vi "Main.vi"() -> ()   [LabVIEW 2014, in "GenNet-Server.lvlib"]
doc: "The GenNet-Server module is instantiated from a DQMH Generic Networking Module\nin order to accept messages via TCP/IP. \n\nThe GenNet-Server module accepts messages from any DQMH Generic Networking \nModule running in another application and/or on another PC.\n\n<b>Note:</b> This VI was modified by the <b>Validate DQMH Module</b> tool to upgrade it to the DQMH 5.0 approach to destroying cloneable module event references.\n\n<b>Note:</b> This VI was modified by the <b>Validate DQMH Module</b> tool to have the module name be passed as the Additional Information parameter with an Error Reported broadcast.\n\n<b>Note:</b> This VI was modified by the <b>Validate DQMH Module</b> tool to call the Release Message Queue VI in the top-level Error case.\n\n<b>Note:</b> This VI was modified by the <b>Validate DQMH Module</b> tool to call the Release Message Queue VI in the top-level Error case."
uses:
  GenNet-Server.lvlib
  <vilib>/Delacor/Delacor QMH/Libraries/Cloneable Module Admin_class/Delacor_lib_QMH_Cloneable Module Admin.lvclass
  DQMH-GenNet Message Queue.lvclass
  TCP_Comm-States.ctl
  UDP Broadcasting/Generic Broadcasts.ctl
  hse-dqmh/Dynamic Requesters/Singleton/Status Updated Argument--cluster.ctl
  hse-dqmh/Dynamic Requesters/Singleton/Error Reported Argument--cluster.ctl
  hse-dqmh/Dynamic Requesters/Singleton/Get Module Execution Status Argument--cluster.ctl
  hse-dqmh/Dynamic Requesters/Singleton/Stop Argument--cluster.ctl
  hse-dqmh/Controls/System Message Argument--cluster.ctl
  hse-dqmh/Controls/System Message Source.ctl
  Module Data--cluster.ctl
  UDP Broadcasting/Network Broadcast Params.ctl
  Stop Argument--cluster.ctl
  <vilib>/Delacor/Delacor QMH/Libraries/Message Queue_class/Delacor_lib_QMH_Message Queue.lvclass/Delacor_lib_QMH_Message Queue.ctl
  UDP Broadcasting/Broadcast Arguments/Error Reported - Arguments.ctl
  UDP Broadcasting/Broadcast Arguments/Module Did Stop - Arguments.ctl
  Forward Generic Broadcasts to Network Argument--cluster.ctl
  <vilib>/Delacor/Delacor QMH/Libraries/Cloneable Module Admin_class/Delacor_lib_QMH_Cloneable Module Admin.lvclass/Delacor_lib_QMH_Cloneable Module Admin.ctl
  <vilib>/Delacor/Delacor QMH/Libraries/Module Admin_class/Delacor_lib_QMH_Module Admin.lvclass/Delacor_lib_QMH_Module Admin.ctl
  <vilib>/Utility/miscctls.llb/LVPointTypeDef.ctl
  <vilib>/Delacor/Delacor QMH/Libraries/Message Queue_class/Delacor_lib_QMH_Enqueue Message (Single).vi
  <vilib>/Delacor/Delacor QMH/Libraries/Cloneable Module Admin_class/Delacor_lib_QMH_Get Module ID.vi
  <vilib>/Delacor/Delacor QMH/Libraries/Module Admin_class/Delacor_lib_QMH_Get External Launch.vi
  <vilib>/Utility/tcp.llb/UDP Multicast Write-Only Open.vi
  <vilib>/Utility/error.llb/Error Cluster From Error Code.vi
  <vilib>/ErrorRing/Error Ring.xnode
  <vilib>/Delacor/Delacor QMH/Libraries/Message Queue_class/Delacor_lib_QMH_Message Queue.lvclass
  hse-dqmh/hse-dqmh.lvlib
  hse-gennet.lvlib
  hse-dqmh/hse-dqmh-dynamicrequesters.lvlib
panel:
  in  "Call Chain":string[](array[string])
  out "listener ID":refnum<k5>
  in  "Port Number":u16
  in  "Caller MsgQ":refnum<class "DQMH-GenNet Message Queue.lvclass">
  out "error out":errorcluster
  in  "Module Admin":refnum<class "Delacor_lib_QMH_Cloneable Module Admin.lvclass">
  # "The GenNet-Server module is instantiated from a DQMH Generic Networking Module\n(the caller) in order to accept messages via TCP/IP. \n\nThe GenNet-Server module accepts messages from any DQMH Generic Networking \nModule running in another application and/or on another PC."
  # "Caveat:\nThe Caller's message queue, which should be private to the caller only, is avail-\nable to the GenNet-Server module so that it can write messages directly. As the GenNet-Server\nmodule cannot be accessed from other code, and as messages that arrive via\nnetwork are to be considered local, this excemption to the rule is tolerable."
  # "Please get in touch with us at office@hampel-soft.com or visit our website www.hampel-soft.com"
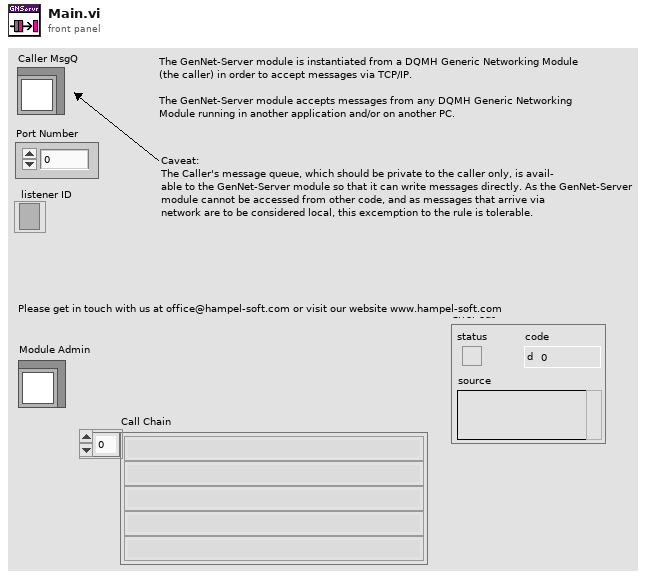
[diagram p1: front panel]
types:
  T1 = typedef "hse-gennet.lvlib/Generic Broadcasts.ctl" = cluster{"Status Updated":refnum<user-event>, "Error Reported":refnum<user-event>, "Update Module Execution Status":refnum<user-event>, "Module Did Stop":refnum<user-event>, "System Message":refnum<user-event>}
  T2 = typedef "GenNet-Server.lvlib/TCP_Comm-States.ctl" = enum16{"Idle", "Open port", "Wait for connection...", "Close port"}
  T3 = typedef "GenNet-Server.lvlib/Request Events--cluster.ctl" = cluster{"Stop Module":refnum<user-event>, "Show Panel":refnum<user-event>, "Hide Panel":refnum<user-event>, "Show Diagram":refnum<user-event>, "Get Module Execution Status":refnum<user-event>, "Forward Generic Broadcasts to Network":refnum<user-event>}
  T4 = typedef "GenNet-Server.lvlib/Module Data--cluster.ctl" = cluster{"Status":string, "UDP Conn. ID":refnum<k16>, "Network Broadcast Params":T5}
  T5 = typedef "hse-gennet.lvlib/Network Broadcast Params.ctl" = cluster{"Server (Sender) Port":u16, "Client (Receiver) Port":u16, "Multicast Address":string, "Local IP Address":string, "Max Rx Byte Size":i32}
  T6 = enum32{"invalid lock state", "Not Locked", "Locked (No Password)", "Password-protected"}
  T7 = typedef "GenNet-Server.lvlib/Stop Argument--cluster.ctl" = cluster{"Origin":string, "Module ID":i32, "Exit via Stop Module Req?":bool, "Wait for Module to stop?":bool}
  T8 = typedef "hse-gennet.lvlib/Error Reported - Arguments.ctl" = cluster{"Error":errorcluster, "Additional Information":string, "Module Name":string}
  T9 = typedef "hse-gennet.lvlib/Module Did Stop - Arguments.ctl" = cluster{"Origin":string, "Exit via Stop Module Req?":bool, "Wait for Module to stop?":bool}
  T10 = typedef "hse-dqmh.lvlib/System Message Source.ctl" = enum16{"module", "application", "network"}
  T11 = typedef "hse-dqmh.lvlib/System Message Argument--cluster.ctl" = cluster{"Identifier":string, "Payload":variant, "Source Type":T10, "Source Name":string}
  T12 = typedef "GenNet-Server.lvlib/Forward Generic Broadcasts to Network Argument--cluster.ctl" = cluster{"Module ID":i32, "Generic Broadcast Events":T1, "Network Broadcast Params":T5}
  T13 = typedef "LVPointTypeDef.ctl" = cluster{"Horizontal":i16, "Vertical":i16}
  T14 = enum32{"Invalid", "Standard", "Closed", "Hidden", "Minimized", "Maximized"}
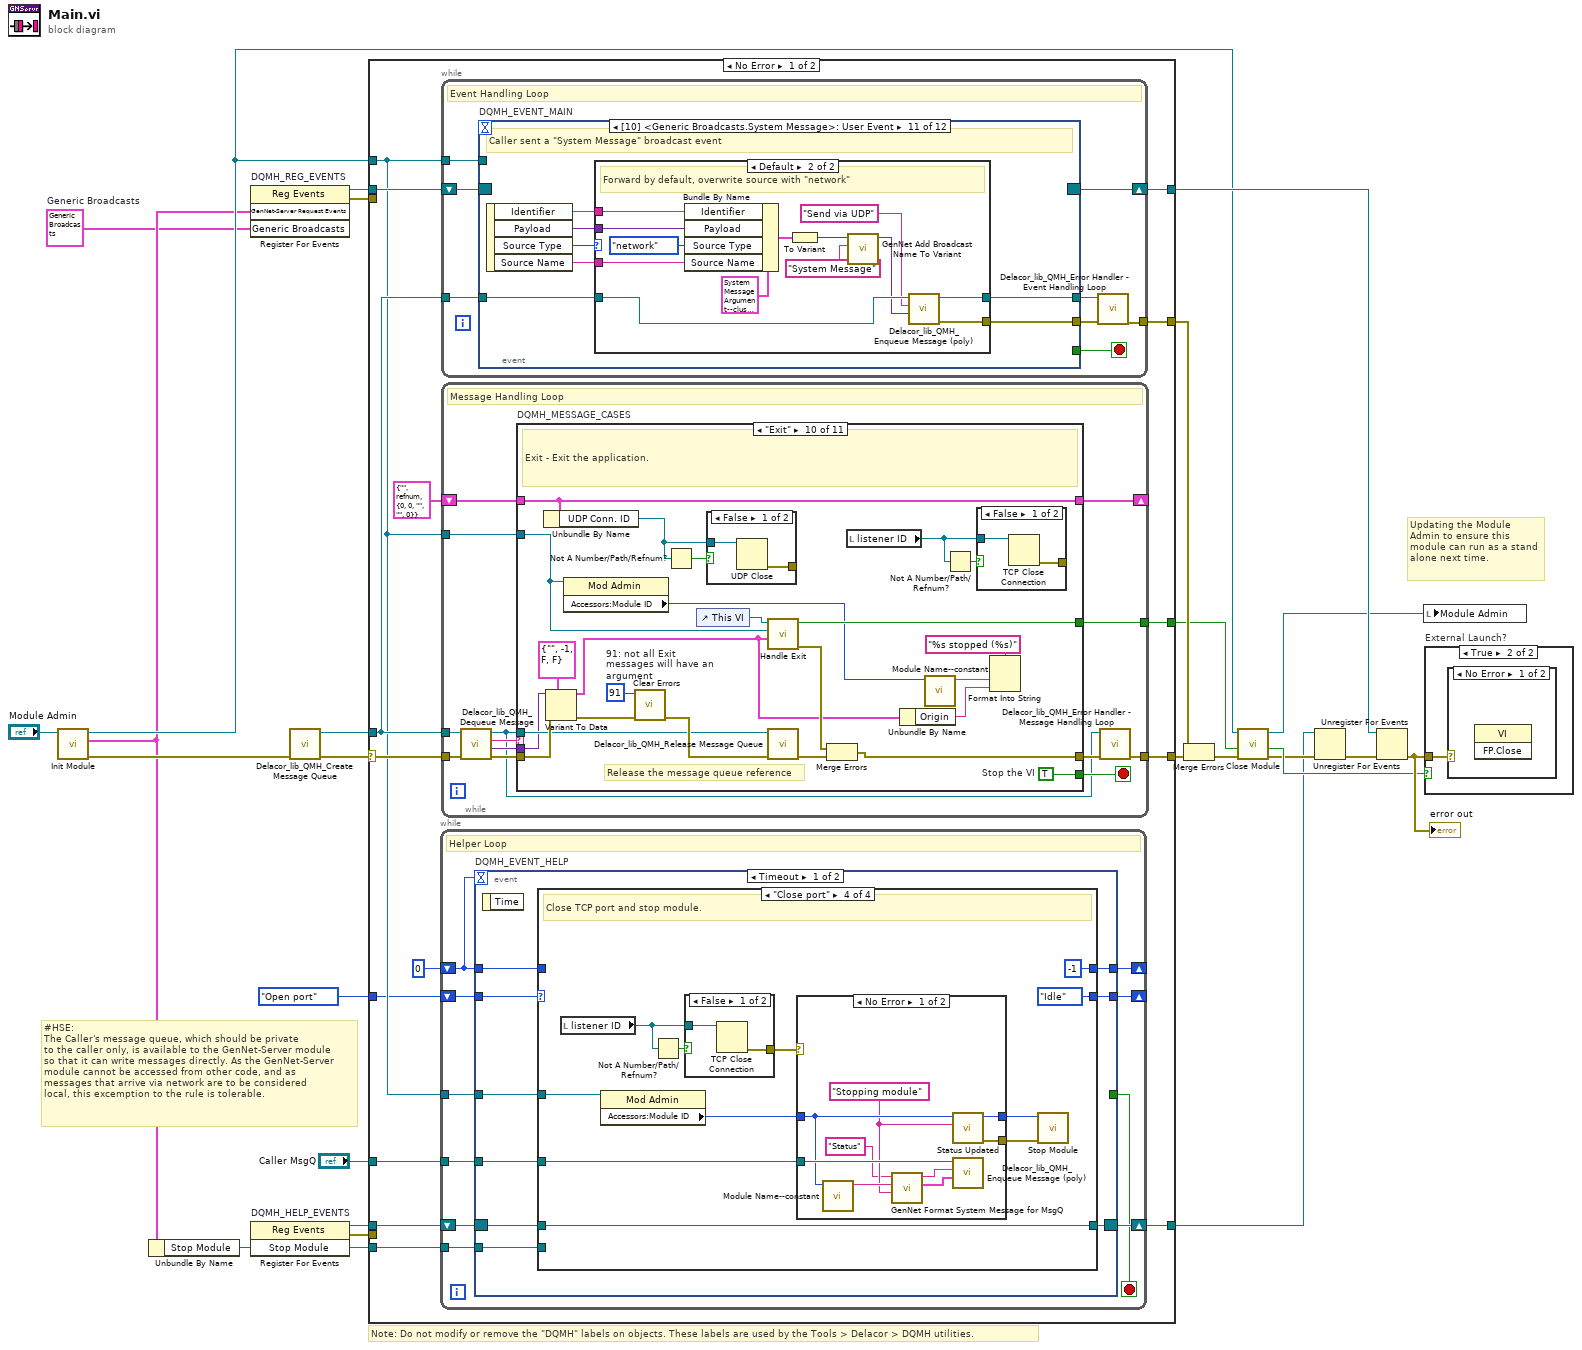
[diagram p0: block diagram]
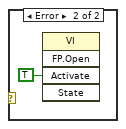
[diagram p3: hidden frame]
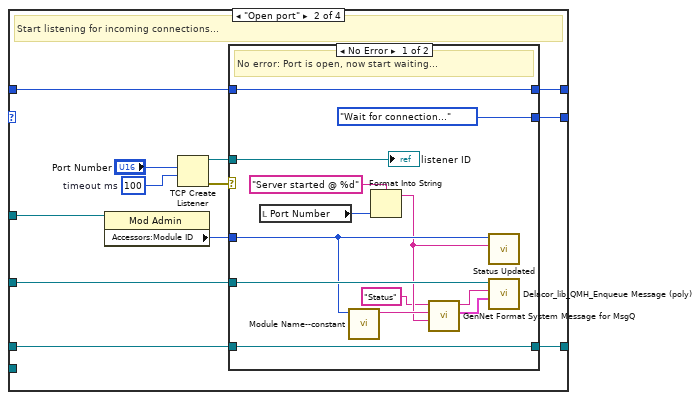
[diagram p5: hidden frame]
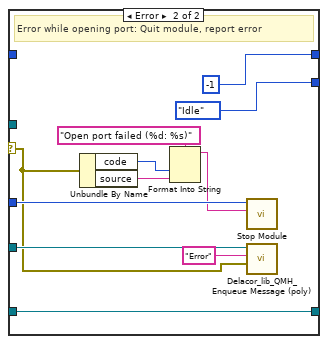
[diagram p6: hidden frame]
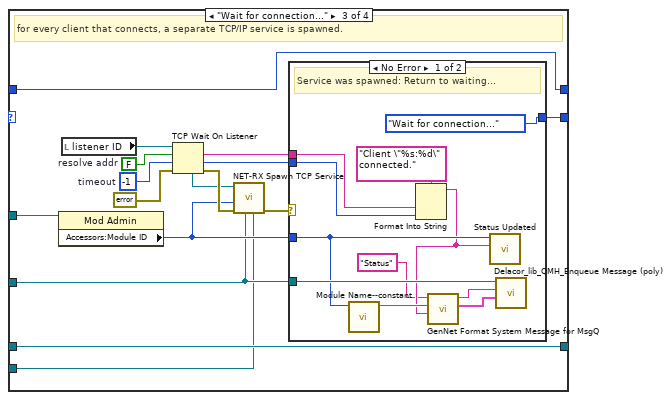
[diagram p7: hidden frame]
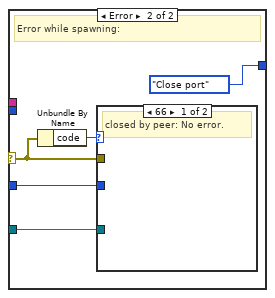
[diagram p8: hidden frame]
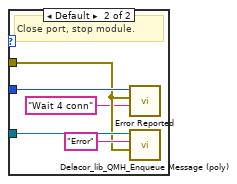
[diagram p9: hidden frame]
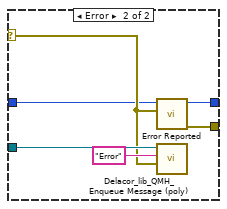
[diagram p11: hidden frame]
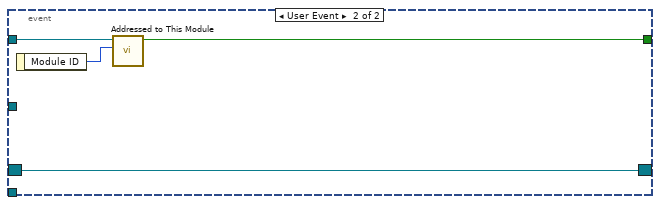
[diagram p12: hidden frame]
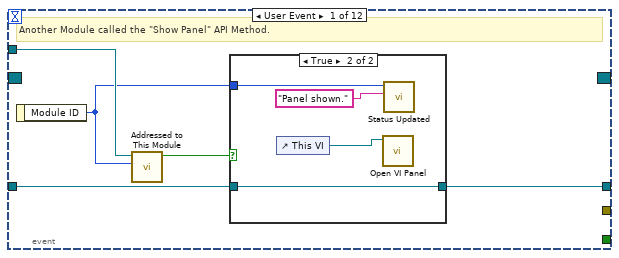
[diagram p13: hidden frame]
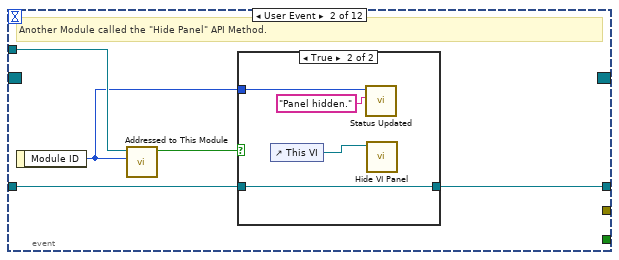
[diagram p15: hidden frame]
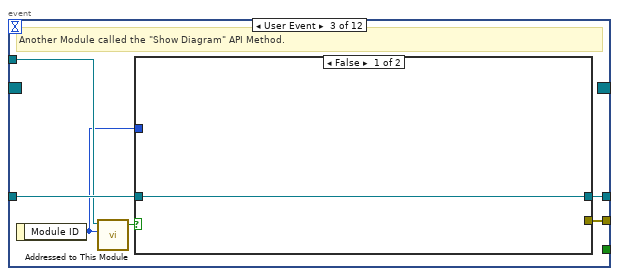
[diagram p17: hidden frame]
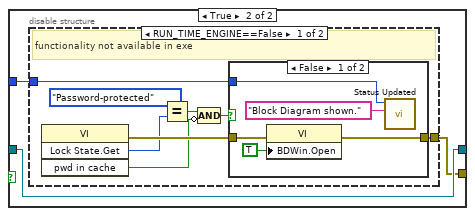
[diagram p18: hidden frame]
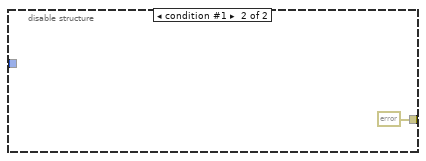
[diagram p20: hidden frame]
diagram:
  w1 = T1 {"Status Updated"=refnum, "Error Reported"=refnum, "Update Module Execution Status"=refnum, "Module Did Stop"=refnum, "System Message"=refnum}  # Generic Broadcasts
  # "#HSE: \nThe Caller's message queue, which should be private \nto the caller only, is available to the GenNet-Server module \nso that it can write messages directly. As the GenNet-Server\nmodule cannot be accessed from other code, and as \nmessages that arrive via network are to be considered \nlocal, this excemption to the rule is tolerable."
  # "Note: Do not modify or remove the \"DQMH\" labels on objects. These labels are used by the Tools > Delacor > DQMH utilities."
  # "Updating the Module Admin to ensure this module can run as a stand alone next time."
  n1 = call "Init Module.vi"("Cloneable Module Admin in"="Module Admin") -> ("error out"=w22:errorcluster, "GenNet-Server Request Events"=w6:T3, "Cloneable Module Admin out"=w17:refnum<class "Delacor_lib_QMH_Cloneable Module Admin.lvclass">)  [unwired: 8 in]
  n2 = Unbundle By Name(w6) -> ("Stop Module"=w5:refnum<user-event>)
  n3 = register-events "DQMH_REG_EVENTS"(w6, w1) -> (reference out=w20:refnum<event-registration>, error out=w3:errorcluster)  [unwired: 2 in]
  n4 = register-events "DQMH_HELP_EVENTS"(w5) -> (reference out=w11:refnum<event-registration>, error out=w2:errorcluster)  [unwired: 2 in]
  n5 = call <vilib>:"Delacor_lib_QMH_Create Message Queue.vi"("error in (no error)"=w22) -> ("error out"=w12:errorcluster, "Message Queue"=w19:refnum<class "Delacor_lib_QMH_Message Queue.lvclass">)  [unwired: 9 in]
  n6 = case shown="No Error" w12 {
    selector: w12 -> [w34 w500]
    tunnel: [w40 w500] -> w23
    tunnel: [w39 w501] -> w21
    tunnel: w20 -> [w37 w501]
    tunnel: w19 -> [w36 w492]
    tunnel: [w35 _] -> w24
    tunnel: w17 -> [w31 w496]
    tunnel: [w33 _] -> w15
    tunnel: w11 -> [w32 w493]
    tunnel: "Caller MsgQ" -> [w30 w491]
    tunnel: [w29 w493] -> w7
    tunnel: w5 -> [w27 _]
    tunnel: TCP_Comm-States."Open port" ("comm-states") -> [w26 _]
    tunnel: w3 -> [_ _]
    tunnel: w2 -> [_ _]
    frame No Error {
      n7 = while {
        shift-right: [w49] -> _
        shift-left: 0 -> [w50]
        tunnel: w31 -> [w48]
        tunnel: w30 -> [w47]
        shift-right: [w44] -> _
        shift-left: w26 -> [w45]
        shift-right: [w46] -> w29
        shift-left: w32 -> [w42]
        tunnel: w27 -> [w41]
        stop <- w43 stop-if-true
        # "Helper Loop"
        n8 = event "DQMH_EVENT_HELP" shown="[0] Timeout" {
          selector: w42 -> [w53 w162]
          dyn-events: [w52 w162] -> w46
          timeout: w50 -> [_ _]
          tunnel: w50 -> [w58 _]
          tunnel: [w57 _] -> w49
          tunnel: w48 -> [w56 w165]
          tunnel: w47 -> [w54 _]
          tunnel: w45 -> [w59 _]
          tunnel: [w55 _] -> w44
          tunnel: [_ w163] -> w43
          tunnel: w41 -> [w51 _]
          event Timeout {
            n9 = event-data() -> ()  [unwired: 1 in, 1 out]
            n10 = case shown="\"Close port\"" w59 {
              selector: w59 -> [w62 _ _ _]
              tunnel: w58 -> [w61 w67 w99 _]
              tunnel: [w61 w66 w99 -1] -> w57
              tunnel: w56 -> [_ w70 w111 w145]
              tunnel: [w62 w74 w106 TCP_Comm-States."Idle" ("comm-states")] -> w55
              tunnel: w54 -> [_ w68 w107 w146]
              tunnel: w53 -> [w60 w65 w105 w139]
              tunnel: [w60 w64 w105 w139] -> w52
              tunnel: w51 -> [_ _ w104 _]
              frame "Idle", Default {
              }
              frame "Open port" {
                w73 = 100  # timeout ms
                # "Start listening for incoming connections..."
                n11 = property class="Mod Admin"(reference=w70) -> ("Accessors:Module ID"=w69:i32)  [unwired: 1 in, 2 out]
                n12 = TCP Create Listener(9:w73, 10:"Port Number") -> (0:w72:errorcluster, 3:w71:refnum<k5>)  [unwired: 3 in, 1 out]
                n13 = case shown="No Error" w72 {
                  selector: w72 -> [_ w88]
                  tunnel: [TCP_Comm-States."Wait for connection..." ("comm-states") TCP_Comm-States."Idle" ("comm-states")] -> w74
                  tunnel: w71 -> [w83 _]
                  tunnel: w69 -> [w78 w93]
                  tunnel: w68 -> [w85 w96]
                  tunnel: w67 -> [w84 _]
                  tunnel: [w84 -1] -> w66
                  tunnel: w65 -> [w82 w94]
                  tunnel: [w82 w94] -> w64
                  frame No Error {
                    # "No error: Port is open, now start waiting..."
                    n14 = local read "Port Number"() -> (w80:u16)
                    n15 = call "Module Name--constant.vi"("Module ID"=w78) -> ("Module Name"=w77:string)  [unwired: 10 in]
                    n16 = Format Into String(format string="Server started @ %d" ("Status"), w80) -> (resulting string=w76:string)  [unwired: 2 in, 1 out]
                    n17 = call "GenNet Format System Message for MsgQ.vi"("Payload"=w76, "Source Name"=w77, "Identifer"="Status") -> ("System Message Argument"=w79:T11, "System Message constant"=w87:string)  [unwired: 7 in]
                    n18 = call "Status Updated.vi"("Status"=w76, "Module ID"=w78) -> ()  [unwired: 9 in, 1 out]
                    n19 = call-poly <vilib>:"Delacor_lib_QMH_Enqueue Message (poly).vi"("Message Data"=w79, "Message"=w87, "Message Queue in"=w85) -> ()  [unwired: 7 in, 2 out]
                    "listener ID" <- w83
                  }
                  frame Error {
                    # "Error while opening port: Quit module, report error"
                    n20 = Unbundle By Name(w88) -> ("code"=w90:i32, "source"=w91:string)
                    n21 = Format Into String(format string="Open port failed (%d: %s)" ("Origin"), w90, w91) -> (resulting string=w89:string)  [unwired: 2 in, 1 out]
                    n22 = call "Stop Module.vi"("Origin"=w89, "Module ID"=w93) -> ()  [unwired: 9 in, 1 out]
                    n23 = call-poly <vilib>:"Delacor_lib_QMH_Enqueue Message (poly).vi"("Message Data"=w88, "Message"="Error", "Message Queue in"=w96) -> ()  [unwired: 7 in, 2 out]
                  }
                }
              }
              frame "Wait for connection..." {
                w101 = FALSE  # resolve addr
                w114 = -1  # timeout
                # "for every client that connects, a separate TCP/IP service is spawned."
                n24 = property class="Mod Admin"(reference=w111) -> ("Accessors:Module ID"=w109:i32)  [unwired: 1 in, 2 out]
                n25 = local read "listener ID"() -> (w108:refnum<k5>)
                n26 = TCP Wait On Listener(8:errorcluster {"status"=FALSE, "code"=0, "source"=""} ("error in (no error)"), 9:w114, 10:w101, 11:w108) -> (0:w113:errorcluster, 1:w102:u16, 2:w103:string, 4:w112:refnum<k5>)  [unwired: 1 out]
                n27 = call "NET-RX Spawn TCP Service.vi"("Stop Module"=w104, "Caller MsgQ"=w107, "error in"=w113, "Module ID"=w109, "Connection ID"=w112) -> ("error out"=w110:errorcluster)  [unwired: 6 in]
                n28 = case shown="No Error" w110 {
                  selector: w110 -> [_ w127]
                  tunnel: w107 -> [w121 w130]
                  tunnel: w109 -> [w118 w129]
                  tunnel: [TCP_Comm-States."Wait for connection..." ("comm-states") TCP_Comm-States."Close port" ("comm-states")] -> w106
                  tunnel: w103 -> [w123 _]
                  tunnel: w102 -> [w122 _]
                  frame No Error {
                    # "Service was spawned: Return to waiting..."
                    n29 = call "Module Name--constant.vi"("Module ID"=w118) -> ("Module Name"=w117:string)  [unwired: 10 in]
                    n30 = Format Into String(format string="Client \"%s:%d\" connected.", w123, w122) -> (resulting string=w116:string)  [unwired: 2 in, 1 out]
                    n31 = call "GenNet Format System Message for MsgQ.vi"("Payload"=w116, "Source Name"=w117, "Identifer"="Status") -> ("System Message Argument"=w120:T11, "System Message constant"=w119:string)  [unwired: 7 in]
                    n32 = call "Status Updated.vi"("Status"=w116, "Module ID"=w118) -> ()  [unwired: 9 in, 1 out]
                    n33 = call-poly <vilib>:"Delacor_lib_QMH_Enqueue Message (poly).vi"("Message Data"=w120, "Message"=w119, "Message Queue in"=w121) -> ()  [unwired: 7 in, 2 out]
                  }
                  frame Error {
                    # "Error while spawning:"
                    n34 = Unbundle By Name(w127) -> ("code"=w126:i32)
                    n35 = case shown="66" w126 {
                      tunnel: w130 -> [_ w135]
                      tunnel: w127 -> [_ w132]
                      tunnel: w129 -> [_ w133]
                      frame 66 {
                        # "closed by peer: No error."
                      }
                      frame Default {
                        # "Close port, stop module."
                        n36 = call "Error Reported.vi"("Additional Information"="Wait 4 conn", "Error"=w132, "Module ID"=w133) -> ()  [unwired: 8 in, 1 out]
                        n37 = call-poly <vilib>:"Delacor_lib_QMH_Enqueue Message (poly).vi"("Message Data"=w132, "Message"="Error", "Message Queue in"=w135) -> ()  [unwired: 7 in, 2 out]
                      }
                    }
                  }
                }
              }
              frame "Close port" {
                # "Close TCP port and stop module."
                n38 = local read "listener ID"() -> (w140:refnum<k5>)
                n39 = property class="Mod Admin"(reference=w145) -> ("Accessors:Module ID"=w138:i32)  [unwired: 1 in, 2 out]
                n40 = Not A Number/Path/Refnum?(number/path/refnum=w140) -> (NaN/Path/Refnum?=w142:bool)
                n41 = case shown="False" w142 {
                  tunnel: [w148 _] -> w141
                  tunnel: w140 -> [w147 _]
                  frame False {
                    n42 = TCP Close Connection(connection ID=w147) -> (error out=w148:errorcluster)  [unwired: 2 in, 1 out]
                  }
                  frame True {
                  }
                }
                n43 = case shown="No Error" w141 {
                  selector: w141 -> [_ w159]
                  tunnel: w146 -> [w155 w160]
                  tunnel: w138 -> [w152 w157]
                  tunnel: [w156 w158] -> w137
                  tunnel: [w152 w157] -> w136
                  frame No Error {
                    w150 = "Stopping module" ("Status")
                    n44 = call "Module Name--constant.vi"("Module ID"=w152) -> ("Module Name"=w151:string)  [unwired: 10 in]
                    n45 = call "GenNet Format System Message for MsgQ.vi"("Payload"=w150, "Source Name"=w151, "Identifer"="Status") -> ("System Message Argument"=w153:T11, "System Message constant"=w154:string)  [unwired: 7 in]
                    n46 = call "Status Updated.vi"("Status"=w150, "Module ID"=w152) -> ("error out"=w156:errorcluster)  [unwired: 9 in]
                    n47 = call-poly <vilib>:"Delacor_lib_QMH_Enqueue Message (poly).vi"("Message Data"=w153, "Message"=w154, "Message Queue in"=w155) -> ()  [unwired: 7 in, 2 out]
                  }
                  frame Error {
                    n48 = call "Error Reported.vi"("Error"=w159, "Module ID"=w157) -> ("error out"=w158:errorcluster)  [unwired: 9 in]
                    n49 = call-poly <vilib>:"Delacor_lib_QMH_Enqueue Message (poly).vi"("Message Data"=w159, "Message"="Error", "Message Queue in"=w160) -> ()  [unwired: 7 in, 2 out]
                  }
                }
                n50 = call "Stop Module.vi"("error in (no error)"=w137, "Module ID"=w136) -> ()  [unwired: 9 in, 1 out]
              }
            }
          }
          event User Event {
            n51 = event-data() -> ("Module ID"=w164:i32)  [unwired: 1 in]
            n52 = call "Addressed to This Module.vi"("Module ID from Argument"=w164, "Module Admin"=w165) -> ("Addressed to this instance?"=w163:bool)  [unwired: 8 in, 1 out]
          }
        }
      }
      n53 = while {
        tunnel: w36 -> [w173]
        shift-right: [w171] -> w39
        shift-left: w37 -> [w172]
        tunnel: [w167] -> w35
        tunnel: w31 -> [w166]
        stop <- w169 stop-if-true
        # "Event Handling Loop"
        n54 = event "DQMH_EVENT_MAIN" shown="[10] <Generic Broadcasts.System Message>: User Event" {
          selector: w172 -> [_ _ _ _ _ _ _ _ _ _ _ w318]
          dyn-events: [_ _ _ _ _ _ _ _ _ _ _ w319] -> w171
          timeout: _ -> [_ _ _ _ _ _ _ _ _ _ _ _]
          tunnel: [_ _ _ w222 _ _ _ _ _ _ _ _] -> w169
          tunnel: w173 -> [w178 w188 w199 w225 w245 w249 w261 w274 w280 w293 w301 w325]
          tunnel: [_ _ w194 w227 w244 w248 w259 w271 w279 w291 w299 w321] -> w170
          tunnel: [w177 w187 w198 w226 w243 w249 w260 w272 w281 w292 w300 w324] -> w168
          tunnel: w166 -> [w175 w185 w196 w224 _ w250 _ _ _ _ _ w322]
          event User Event {
            # "Another Module called the \"Show Panel\" API Method."
            n55 = event-data() -> ("Module ID"=w174:i32)  [unwired: 1 in]
            n56 = call "Addressed to This Module.vi"("Module ID from Argument"=w174, "Module Admin"=w175) -> ("Addressed to this instance?"=w176:bool)  [unwired: 8 in, 1 out]
            n57 = case shown="True" w176 {
              tunnel: w178 -> [w179 w183]
              tunnel: [w179 w183] -> w177
              tunnel: w174 -> [_ w181]
              frame False {
              }
              frame True {
                n58 = control-ref of="This VI"() -> (w180:refnum<vi>)
                n59 = call "Open VI Panel.vi"("VI"=w180) -> ()  [unwired: 10 in, 1 out]
                n60 = call "Status Updated.vi"("Status"="Panel shown." ("format string"), "Module ID"=w181) -> ()  [unwired: 9 in, 1 out]
              }
            }
          }
          event User Event {
            # "Another Module called the \"Hide Panel\" API Method."
            n61 = event-data() -> ("Module ID"=w184:i32)  [unwired: 1 in]
            n62 = call "Addressed to This Module.vi"("Module ID from Argument"=w184, "Module Admin"=w185) -> ("Addressed to this instance?"=w186:bool)  [unwired: 8 in, 1 out]
            n63 = case shown="True" w186 {
              tunnel: w188 -> [w189 w193]
              tunnel: [w189 w193] -> w187
              tunnel: w184 -> [_ w191]
              frame False {
              }
              frame True {
                n64 = control-ref of="This VI"() -> (w190:refnum<vi>)
                n65 = call "Status Updated.vi"("Status"="Panel hidden." ("format string"), "Module ID"=w191) -> ()  [unwired: 9 in, 1 out]
                n66 = call "Hide VI Panel.vi"("VI"=w190) -> ()  [unwired: 10 in, 1 out]
              }
            }
          }
          event User Event {
            # "Another Module called the \"Show Diagram\" API Method."
            n67 = event-data() -> ("Module ID"=w195:i32)  [unwired: 1 in]
            n68 = call "Addressed to This Module.vi"("Module ID from Argument"=w195, "Module Admin"=w196) -> ("Addressed to this instance?"=w197:bool)  [unwired: 8 in, 1 out]
            n69 = case shown="False" w197 {
              tunnel: w199 -> [w200 w202]
              tunnel: [w200 w202] -> w198
              tunnel: w195 -> [_ w203]
              tunnel: [_ w201] -> w194
              frame False {
              }
              frame True {
                n70 = disable-structure shown="RUN_TIME_ENGINE==False" {
                  disable-tunnel: [w211 errorcluster {"status"=FALSE, "code"=0, "source"=""} ("error out")] -> w201
                  disable-tunnel: w203 -> [w204 _]
                  frame condition #0 (active) {
                    # "functionality not available in exe"
                    n71 = invoke class="VI" method="Lock State.Get"() -> (error out=w210:errorcluster, "Get Lock State"=w209:T6, "pwd in cache"=w206:bool)  [unwired: 4 in, 1 out]
                    n72 = Equal?(x=T6."Password-protected", y=w209) -> (x = y?=w207:bool)
                    n73 = Compound Arithmetic op=AND(w207, invert w206) -> (w205:bool)
                    n74 = case shown="False" w205 {
                      tunnel: [w215 w217] -> w211
                      tunnel: w210 -> [w214 w217]
                      tunnel: w204 -> [w212 _]
                      frame False {
                        n75 = property class="VI"(error in=w214, "BDWin.Open"=TRUE ("Block Diagram Window:Open")) -> (error out=w215:errorcluster)  [unwired: 1 in, 1 out]
                        n76 = call "Status Updated.vi"("Status"="Block Diagram shown." ("format string"), "Module ID"=w212) -> ()  [unwired: 9 in, 1 out]
                      }
                      frame True {
                        # "Password-protected VI, and the password is not in the cache. Do not show the diagram."
                      }
                    }
                  }
                  frame condition #1 {
                  }
                }
              }
            }
          }
          event User Event {
            # "Another Module called the \"Stop Module\" API Method  or the Message Handling Loop below."
            n77 = event-data() -> ("Module ID"=w220:i32, "Wait for Module to stop?"=w221:bool, "Origin"=w219:string)  [unwired: 1 in]
            n78 = call "Addressed to This Module.vi"("Module ID from Argument"=w220, "Module Admin"=w224) -> ("Addressed to this instance?"=w223:bool)  [unwired: 8 in, 1 out]
            n79 = case shown="True" w223 {
              tunnel: [_ w237] -> w227
              tunnel: [w228 w236] -> w226
              tunnel: w225 -> [w228 w235]
              tunnel: [_ TRUE] -> w222
              tunnel: w221 -> [_ w230]
              tunnel: w220 -> [_ w232]
              tunnel: w219 -> [_ _]
              frame False {
              }
              frame True {
                # "The event can get fired from the Exit message. The queue gets destroyed there. In this case, the Enqueue VI will return error 1. It is safe to ignore, because the module is already exiting."
                n80 = Bundle By Name(cluster=T7 {"Origin"="", "Module ID"=-1, "Exit via Stop Module Req?"=FALSE, "Wait for Module to stop?"=FALSE} ("Stop Argument"), "Module ID"=w232, "Exit via Stop Module Req?"=TRUE, "Wait for Module to stop?"=w230) -> (w229:T7)
                n81 = call-poly <vilib>:"Delacor_lib_QMH_Enqueue Message (poly).vi"("Priority Message? (F)"=TRUE, "Message Data"=w229, "Message"="Exit", "Message Queue in"=w235) -> ("error out"=w240:errorcluster, "Message Queue out"=w236:refnum<class "Delacor_lib_QMH_Message Queue.lvclass">)  [unwired: 6 in]
                n82 = call <vilib>:"Clear Errors.vi"("error in (no error)"=w240, "specific error code to clear (0: all)"=1) -> ("error out"=w237:errorcluster)  [unwired: 4 in, 1 out]
              }
            }
          }
          event Panel Close? {
            w246 = TRUE  # Discard the event so the 'Confirm Quit' message has a chance to run.
            # "Send the 'Confirm Quit' message if the user closes the panel of the VI."
            n83 = event-data() -> ()  [unwired: 1 in, 1 out]
            n84 = call-poly <vilib>:"Delacor_lib_QMH_Enqueue Message (poly).vi"("Message"="Confirm Quit", "Message Queue in"=w245) -> ("error out"=w244:errorcluster, "Message Queue out"=w243:refnum<class "Delacor_lib_QMH_Message Queue.lvclass">)  [unwired: 8 in]
            n85 = event-data("Discard?"=w246) -> ()  [unwired: 1 in, 1 out]
          }
          event User Event {
            # "For cloneable running as singleton, broadcast that the module is running."
            n86 = event-data() -> ("Module ID"=w247:i32)  [unwired: 1 in]
            n87 = call "Addressed to This Module.vi"("Module ID from Argument"=w247, "Module Admin"=w250) -> ("Addressed to this instance?"=w251:bool)  [unwired: 8 in, 1 out]
            n88 = case shown="True" w251 {
              tunnel: [_ w254] -> w248
              tunnel: w247 -> [_ w253]
              frame False {
              }
              frame True {
                n89 = call "Update Module Execution Status.vi"("Running?"=TRUE, "Module ID"=w253) -> ("error out"=w254:errorcluster)  [unwired: 9 in]
              }
            }
          }
          event User Event {
            # "Caller sent a \"Status Updated\" broadcast event"
            n90 = event-data() -> ("Status"=w256:string)  [unwired: 1 in]
            n91 = To Variant(anything=w256) -> (Variant=w258:variant)
            n92 = call "GenNet Add Broadcast Name To Variant.vi"("Broadcast Name"="Status Updated", "Broadcast Data IN"=w258) -> ("Variant OUT"=w255:variant)  [unwired: 9 in]
            n93 = call-poly <vilib>:"Delacor_lib_QMH_Enqueue Message (poly).vi"("Message Data"=w255, "Message"="Send via UDP", "Message Queue in"=w261) -> ("error out"=w259:errorcluster, "Message Queue out"=w260:refnum<class "Delacor_lib_QMH_Message Queue.lvclass">)  [unwired: 7 in]
          }
          event User Event {
            # "Caller sent a \"Error reported\" broadcast event"
            n94 = event-data() -> ("Error"=w269:errorcluster, "Additional Information"=w268:string, "Module Name"=w267:string)  [unwired: 1 in]
            n95 = Bundle By Name(cluster=T8 {"Error"={"status"=FALSE, "code"=0, "source"=""}, "Additional Information"="", "Module Name"=""}, "Error"=w269, "Additional Information"=w268, "Module Name"=w267) -> (w264:T8)
            n96 = To Variant(anything=w264) -> (Variant=w266:variant)
            n97 = call "GenNet Add Broadcast Name To Variant.vi"("Broadcast Name"="Error Reported", "Broadcast Data IN"=w266) -> ("Variant OUT"=w263:variant)  [unwired: 9 in]
            n98 = call-poly <vilib>:"Delacor_lib_QMH_Enqueue Message (poly).vi"("Message Data"=w263, "Message"="Send via UDP", "Message Queue in"=w274) -> ("error out"=w271:errorcluster, "Message Queue out"=w272:refnum<class "Delacor_lib_QMH_Message Queue.lvclass">)  [unwired: 7 in]
          }
          event User Event {
            # "Caller sent a \"Update Module Execution Status\" broadcast event"
            n99 = event-data() -> ("Running?"=w276:bool)  [unwired: 1 in]
            n100 = To Variant(anything=w276) -> (Variant=w278:variant)
            n101 = call "GenNet Add Broadcast Name To Variant.vi"("Broadcast Name"="Update Module Execution Status", "Broadcast Data IN"=w278) -> ("Variant OUT"=w275:variant)  [unwired: 9 in]
            n102 = call-poly <vilib>:"Delacor_lib_QMH_Enqueue Message (poly).vi"("Message Data"=w275, "Message"="Send via UDP", "Message Queue in"=w280) -> ("error out"=w279:errorcluster, "Message Queue out"=w281:refnum<class "Delacor_lib_QMH_Message Queue.lvclass">)  [unwired: 7 in]
          }
          event User Event {
            # "Caller sent a \"Module Did Stop\" broadcast event"
            n103 = event-data() -> ("Origin"=w290:string, "Exit via Stop Module Req?"=w288:bool, "Wait for Module to stop?"=w289:bool)  [unwired: 1 in]
            n104 = Bundle By Name(cluster=T9 {"Origin"="", "Exit via Stop Module Req?"=FALSE, "Wait for Module to stop?"=FALSE} ("Module Did Stop - Arguments"), "Origin"=w290, "Exit via Stop Module Req?"=w288, "Wait for Module to stop?"=w289) -> (w284:T9)
            n105 = To Variant(anything=w284) -> (Variant=w287:variant)
            n106 = call "GenNet Add Broadcast Name To Variant.vi"("Broadcast Name"="Module Did Stop", "Broadcast Data IN"=w287) -> ("Variant OUT"=w283:variant)  [unwired: 9 in]
            n107 = call-poly <vilib>:"Delacor_lib_QMH_Enqueue Message (poly).vi"("Message Data"=w283, "Message"="Send via UDP", "Message Queue in"=w293) -> ("error out"=w291:errorcluster, "Message Queue out"=w292:refnum<class "Delacor_lib_QMH_Message Queue.lvclass">)  [unwired: 7 in]
          }
          event User Event {
            # "Caller sent a \"System Message\" broadcast event"
            n108 = event-data() -> ("Identifier"=w298:string, "Payload"=w297:variant, "Source Type"=w296:T10, "Source Name"=w295:string)  [unwired: 1 in]
            n109 = case shown="Default" w296 {
              tunnel: w301 -> [w302 w315]
              tunnel: [w302 w313] -> w300
              tunnel: [_ w312] -> w299
              tunnel: w298 -> [_ w311]
              tunnel: w297 -> [_ w310]
              tunnel: w295 -> [_ w304]
              frame "network" {
                # "Do not forward if originally received via network"
              }
              frame Default {
                # "Forward by default, overwrite source with \"network\""
                n110 = Bundle By Name(cluster=T11 {"Identifier"="", "Payload"=variant, "Source Type"=enum."module", "Source Name"=""} ("System Message Argument"), "Identifier"=w311, "Payload"=w310, "Source Type"=System_Message_Source."network" ("Source"), "Source Name"=w304) -> (w309:T11)
                n111 = To Variant(anything=w309) -> (Variant=w308:variant)
                n112 = call "GenNet Add Broadcast Name To Variant.vi"("Broadcast Name"="System Message", "Broadcast Data IN"=w308) -> ("Variant OUT"=w307:variant)  [unwired: 9 in]
                n113 = call-poly <vilib>:"Delacor_lib_QMH_Enqueue Message (poly).vi"("Message Data"=w307, "Message"="Send via UDP", "Message Queue in"=w315) -> ("error out"=w312:errorcluster, "Message Queue out"=w313:refnum<class "Delacor_lib_QMH_Message Queue.lvclass">)  [unwired: 7 in]
              }
            }
          }
          event User Event {
            # "Another Module called the \"Forward Generic Broadcasts to Network\" API Method."
            n114 = event-data() -> ("Generic Broadcast Events"=w317:T1, "Network Broadcast Params"=w316:T5, "Module ID"=w320:i32)  [unwired: 1 in]
            n115 = call "Addressed to This Module.vi"("Module ID from Argument"=w320, "Module Admin"=w322) -> ("Addressed to this instance?"=w323:bool)  [unwired: 8 in, 1 out]
            n116 = case shown="True" w323 {
              tunnel: w325 -> [w327 w337]
              tunnel: [w327 w336] -> w324
              tunnel: [_ w334] -> w321
              tunnel: [w326 w333] -> w319
              tunnel: w318 -> [w326 w332]
              tunnel: w317 -> [_ w331]
              tunnel: w316 -> [_ w330]
              frame False {
              }
              frame True {
                n117 = Bundle By Name(cluster=T12 {"Module ID"=-1, "Generic Broadcast Events"={"Status Updated"=refnum, "Error Reported"=refnum, "Update Module Execution Status"=refnum, "Module Did Stop"=refnum, "System Message"=refnum}, "Network Broadcast Params"={"Server (Sender) Port"=0, "Client (Receiver) Port"=0, "Multicast Address"="", "Local IP Address"="", "Max Rx Byte Size"=0}} ("Forward Generic Broadcasts to Network Argument"), "Network Broadcast Params"=w330) -> (w329:T12)
                n118 = register-events "DQMH_REG_INNER"(reference=w332, w331) -> (reference out=w333:refnum<event-registration>)  [unwired: 2 in, 1 out]
                n119 = call-poly <vilib>:"Delacor_lib_QMH_Enqueue Message (poly).vi"("Message Data"=w329, "Message"="Create UDP Sender", "Message Queue in"=w337) -> ("error out"=w334:errorcluster, "Message Queue out"=w336:refnum<class "Delacor_lib_QMH_Message Queue.lvclass">)  [unwired: 7 in]
              }
            }
          }
        }
        n120 = call-dynamic "Delacor_lib_QMH_Error Handler - Event Handling Loop.vi"("error in (no error)"=w170, "Message Queue in"=w168) -> ("dup error in"=w167:errorcluster)  [unwired: 8 in, 1 out]
      }
      n121 = while {
        tunnel: w36 -> [w342]
        shift-right: [w348] -> _
        shift-left: T4 {"Status"="", "UDP Conn. ID"=refnum, "Network Broadcast Params"={"Server (Sender) Port"=0, "Client (Receiver) Port"=0, "Multicast Address"="", "Local IP Address"="", "Max Rx Byte Size"=0}} ("Data Cluster") -> [w349]
        tunnel: w34 -> [w346]
        tunnel: [w340] -> w40
        tunnel: w31 -> [w339]
        tunnel: [w338] -> w33
        stop <- w347 stop-if-true
        # "Message Handling Loop"
        n122 = call-dynamic "Delacor_lib_QMH_Dequeue Message.vi"("error in (no error)"=w346, "Message Queue in"=w342) -> ("error out"=w345:errorcluster, "Message Data"=w343:variant, "Message"=w344:string, "Message Queue out"=w341:refnum<class "Delacor_lib_QMH_Message Queue.lvclass">)  [unwired: 6 in]
        n123 = case "DQMH_MESSAGE_CASES" shown="\"Exit\"" w344 {
          selector: w344 -> [_ _ _ _ _ _ _ _ _ _ w480]
          tunnel: w341 -> [_ _ _ _ _ _ _ w427 w445 w470 _]
          tunnel: w345 -> [w366 w379 w386 w401 w417 w420 w423 w436 w444 w472 _]
          tunnel: [w351 w377 w394 w403 w415 w418 w421 w426 w443 w449 w481] -> w350
          tunnel: w349 -> [w365 w378 w392 w402 w416 w419 w422 w435 w448 w451 w482]
          tunnel: [w365 w378 w391 w402 w416 w419 w422 w435 w448 w451 w482] -> w348
          tunnel: [_ _ _ _ _ _ _ _ _ w469 _] -> w347
          tunnel: w343 -> [_ _ w384 w400 _ _ _ w434 _ w464 _]
          tunnel: w339 -> [w361 _ _ _ _ _ _ w431 _ w454 w478]
          tunnel: [_ _ _ _ _ _ _ _ _ w462 _] -> w338
          frame "Initialize" {
            # "\"Create UDP Sender\""
            # "Initialize - Any operation that needs to be done before the module can receive messages. Synchronize Caller Events.vi will inform Start Module.vi that the module has launched and is ready to receive messages. Module Did Init.vi will broadcast that the module initialized."
            n124 = call "Synchronize Caller Events.vi"("error in (no error)"=w366, "Module Admin"=w361) -> ("error out"=w363:errorcluster, "Module Admin out"=w360:refnum<class "Delacor_lib_QMH_Cloneable Module Admin.lvclass">)  [unwired: 8 in]
            n125 = property class="Mod Admin"(reference=w360) -> ("Accessors:Module ID"=w359:i32, "Accessors:External Launch"=w362:bool)  [unwired: 1 in, 2 out]
            n126 = call "Module Name--constant.vi"("Module ID"=w359) -> ("Module Name"=w352:string)  [unwired: 10 in]
            n127 = disable-structure shown="TARGET_TYPE==Windows||EMBEDDED_UI==True" {
              disable-tunnel: w362 -> [w369 _]
              disable-tunnel: w352 -> [w367 _]
              frame condition #0 (active) {
                n128 = property class="VI"("Front Panel.Title"=w367) -> (reference out=w375:refnum<vi>, error out=w376:errorcluster)  [unwired: 2 in]
                n129 = Select(t=T14."Hidden" ("State"), s=w369, f=T14."Standard" ("State")) -> (s? t:f=w370:T14)
                n130 = invoke class="VI" method="FP.Open"(reference=w375, error in=w376, "State"=w370) -> (reference out=w374:refnum<vi>, error out=w373:errorcluster)  [unwired: 2 in, 3 out]
                n131 = invoke class="VI" method="FP.Center"(reference=w374, error in=w373) -> ()  [unwired: 1 in, 3 out]
                n132 = property on="Pane" class="Pane"("Origin"=T13 {"Horizontal"=0, "Vertical"=0}) -> ()  [unwired: 2 in, 2 out]
              }
              frame condition #1 {
              }
            }
            n133 = call "Module Did Init.vi"("error in (no error)"=w363, "Initialized?"=TRUE, "Origin"=w352, "Module ID"=w359) -> ("error out"=w351:errorcluster)  [unwired: 7 in]
            n134 = Reverse 1D Array(array="Call Chain") -> (reversed array=w355:string[])
            n135 = Index Array(array=w355) -> (element=w356:string)  [unwired: 1 in]
            n136 = Match Pattern(string=w356, regular expression=".lvlib") -> (before substring=w353:string)  [unwired: 1 in, 3 out]
            n137 = Format Into String(format string="%s initialised from %s", w352, w353) -> ()  [unwired: 2 in, 2 out]
          }
          frame "--- UDP Broadcasting ---" {
            # "Separator -- The following cases handle UDP broadcasting."
            n138 = Merge Errors(w379) -> (w377:errorcluster)
          }
          frame "Create UDP Sender" {
            # "Opens a UDP multicast socket for broadcast forwarding"
            n139 = Variant To Data(error in=w386, type=T12 {"Module ID"=-1, "Generic Broadcast Events"={"Status Updated"=refnum, "Error Reported"=refnum, "Update Module Execution Status"=refnum, "Module Did Stop"=refnum, "System Message"=refnum}, "Network Broadcast Params"={"Server (Sender) Port"=0, "Client (Receiver) Port"=0, "Multicast Address"="", "Local IP Address"="", "Max Rx Byte Size"=0}} ("Forward Generic Broadcasts to Network Argument"), Variant=w384) -> (data=w383:T12, error out=w385:errorcluster)
            n140 = Unbundle By Name(w383) -> ("Network Broadcast Params.Local IP Address"=w380:string, "Network Broadcast Params.Server (Sender) Port"=w387:u16)
            n141 = Unbundle By Name(w383) -> ("Network Broadcast Params"=w382:T5)
            n142 = String To IP(1:w380) -> (0:w393:u32)
            n143 = call-poly <vilib>:"UDP Multicast Open.vi"("net address"=w393, "error in (no error)"=w385, "port"=w387) -> ("error out"=w389:errorcluster, "connection ID"=w390:refnum<k16>)  [unwired: 7 in]
            n144 = Bundle By Name(cluster=w392, "Network Broadcast Params"=w382, "UDP Conn. ID"=w390) -> (w391:T4)
            n145 = Format Into String(format string="Create UDP Sender on Port %d" ("Message"), w387) -> ()  [unwired: 2 in, 2 out]
            n146 = Merge Errors(w389) -> (w394:errorcluster)
          }
          frame "Send via UDP" {
            # "Forwards the broadcast events of the caller via UDP"
            n147 = Unbundle By Name(w402) -> ("Network Broadcast Params.Multicast Address"=w396:string, "Network Broadcast Params.Client (Receiver) Port"=w395:u16, "UDP Conn. ID"=w398:refnum<k16>)
            n148 = Not A Number/Path/Refnum?(number/path/refnum=w398) -> (NaN/Path/Refnum?=w397:bool)
            n149 = case shown="True" w397 {
              tunnel: w401 -> [w413 w414]
              tunnel: [w404 w414] -> w399
              tunnel: w398 -> [w411 _]
              tunnel: w396 -> [w407 _]
              tunnel: w395 -> [w406 _]
              tunnel: w400 -> [w410 _]
              frame False {
                # "Send via UDP"
                n150 = call "GenNet Send UDP Message.vi"("Multicast IP Address"=w407, "timeout [ms]"=1000, "Receiver Port"=w406, "error in (no error)"=w413, "Message Data"=w410, "UDP Network Connection in"=w411) -> ("error out"=w405:errorcluster)  [unwired: 4 in, 1 out]
                n151 = call "GenNet Get Broadcast Name From Variant.vi"("error in"=w405, "Broadcast Data IN"=w410) -> ("error out"=w404:errorcluster, "Broadcast Name"=w408:string)  [unwired: 7 in, 1 out]
                n152 = Format Into String(format string="Send Broadcast \"%s\" via UDP to IP %s and Port %d" ("Message"), w408, w407, w406) -> ()  [unwired: 2 in, 2 out]
              }
              frame True {
                (unwired) "Send via UDP: Invalid UDP Connection ID" ("Message")
                # "Invalid ID"
              }
            }
            n153 = Merge Errors(w399) -> (w403:errorcluster)
          }
          frame "--- Module Specific ---" {
            # "Separator -- The following cases handle messages specific to this Module."
            n154 = Merge Errors(w417) -> (w415:errorcluster)
          }
          frame "---Copy This Frame---" {
            # "Duplicate this frame when creating new messages.  Change this comment in the duplicated frame to describe this message."
            n155 = Merge Errors(w420) -> (w418:errorcluster)
          }
          frame "--- Exit and Error Handling---" {
            # "Separator - the following cases handle errors and exit messages."
            n156 = Merge Errors(w423) -> (w421:errorcluster)
          }
          frame "Error" {
            # "Error - Check the error message data and respond accordingly. This message is sent by the \"Error Handler\" VIs at the end of each loop in this application."
            n157 = property class="Mod Admin"(reference=w431) -> ("Accessors:External Launch"=w428:bool, "Accessors:Module ID"=w430:i32)  [unwired: 1 in, 2 out]
            n158 = Variant To Data(error in=w436, type=errorcluster {"status"=FALSE, "code"=0, "source"=""} ("error constant"), Variant=w434) -> (data=w425:errorcluster, error out=w432:errorcluster)
            n159 = call "Module Name--constant.vi"("Module ID"=w430) -> ("Module Name"=w424:string)  [unwired: 10 in]
            n160 = call "Error Reported.vi"("Additional Information"=w424, "Error"=w425, "Module ID"=w430) -> ()  [unwired: 8 in, 1 out]
            n161 = case shown="False" w428 {
              tunnel: [w441 _] -> w429
              tunnel: w427 -> [w440 _]
              tunnel: w425 -> [w437 _]
              frame False {
                # "If the module is running standalone, then pop up an error dialog and call the \"Exit\" message."
                n162 = call <vilib>:"Simple Error Handler.vi"("error in (no error)"=w437) -> ()  [unwired: 4 in, 5 out]
                n163 = call-poly <vilib>:"Delacor_lib_QMH_Enqueue Message (poly).vi"("Priority Message? (F)"=TRUE, "Message"="Exit", "Message Queue in"=w440) -> ("error out"=w441:errorcluster)  [unwired: 7 in, 1 out]
              }
              frame True {
                # "If the module was launched externally, calling the Error Reported broadcast VI is the only action performed by the \"Error\" message. The module's caller can then process the error appropriately."
              }
            }
            n164 = Merge Errors(w432, w429) -> (w426:errorcluster)
            n165 = local write "error out"(w426) -> ()
          }
          frame "Confirm Quit" {
            # "#CodeNeeded - If you want to provide an \"Are you sure\" dialog (or some other notification) before the application exits, place that code here. This message is typically sent from a Panel Close? event."
            # "Confirm Quit - Message that can confirm whether or not the user wants to exit this instance."
            n166 = call-poly <vilib>:"Delacor_lib_QMH_Enqueue Message (poly).vi"("Priority Message? (F)"=TRUE, "error in (no error)"=w444, "Message"="Exit", "Message Queue in"=w445) -> ("error out"=w447:errorcluster)  [unwired: 6 in, 1 out]
            n167 = Merge Errors(w447) -> (w443:errorcluster)
          }
          frame "Exit" {
            w466 = 91  # 91: not all Exit messages will have an argument
            w469 = TRUE  # Stop the VI
            # "Release the message queue reference"
            # "Exit - Exit the application."
            n168 = Unbundle By Name(w451) -> ("UDP Conn. ID"=w450:refnum<k16>)
            n169 = Variant To Data(error in=w472, type=T7 {"Origin"="", "Module ID"=-1, "Exit via Stop Module Req?"=FALSE, "Wait for Module to stop?"=FALSE} ("Stop Argument"), Variant=w464) -> (data=w458:T7, error out=w465:errorcluster)
            n170 = property class="Mod Admin"(reference=w454) -> ("Accessors:Module ID"=w453:i32)  [unwired: 1 in, 2 out]
            n171 = call <vilib>:"Clear Errors.vi"("error in (no error)"=w465, "specific error code to clear (0: all)"=w466) -> ("error out"=w471:errorcluster)  [unwired: 4 in, 1 out]
            n172 = Not A Number/Path/Refnum?(number/path/refnum=w450) -> (NaN/Path/Refnum?=w452:bool)
            n173 = control-ref of="This VI"() -> (w461:refnum<vi>)
            n174 = case shown="False" w452 {
              tunnel: w450 -> [w474 _]
              tunnel: [w473 _] -> _
              frame False {
                n175 = UDP Close(connection ID=w474) -> (error out=w473:errorcluster)  [unwired: 1 in, 1 out]
              }
              frame True {
              }
            }
            n176 = call "Handle Exit.vi"("Stop Argument"=w458, "Module Admin in"=w454, "VI reference"=w461) -> ("error out"=w467:errorcluster, "Wait for Stop?"=w462:bool)  [unwired: 7 in]
            n177 = call-dynamic "Delacor_lib_QMH_Release Message Queue.vi"("error in (no error)"=w471, "Message Queue"=w470) -> ("error out"=w468:errorcluster)  [unwired: 9 in]
            n178 = Merge Errors(w467, w468) -> (w449:errorcluster)
            n179 = local read "listener ID"() -> (w460:refnum<k5>)
            n180 = Unbundle By Name(w458) -> ("Origin"=w457:string)
            n181 = call "Module Name--constant.vi"("Module ID"=w453) -> ("Module Name"=w456:string)  [unwired: 10 in]
            n182 = Not A Number/Path/Refnum?(number/path/refnum=w460) -> (NaN/Path/Refnum?=w459:bool)
            n183 = case shown="False" w459 {
              tunnel: [w476 _] -> _
              tunnel: w460 -> [w475 _]
              frame False {
                n184 = TCP Close Connection(connection ID=w475) -> (error out=w476:errorcluster)  [unwired: 2 in, 1 out]
              }
              frame True {
              }
            }
            n185 = Format Into String(format string="%s stopped (%s)" ("Message"), w456, w457) -> ()  [unwired: 2 in, 2 out]
          }
          frame Default {
            # "'Default' case only runs if there is a message that isn't defined in any of the other cases.  Output a programming error."
            n186 = property class="Mod Admin"(reference=w478) -> ("Accessors:Module ID"=w477:i32)  [unwired: 1 in, 2 out]
            n187 = call "Module Name--constant.vi"("Module ID"=w477) -> ("Module Name"=w479:string)  [unwired: 10 in]
            n188 = xnode "Error Ring"("parameter 0"=w480, "parameter 1"=w479) -> ("error out"=w481:errorcluster)
          }
        }
        n189 = call-dynamic "Delacor_lib_QMH_Error Handler - Message Handling Loop.vi"("error in (no error)"=w350, "Message Queue in"=w341) -> ("dup error in"=w340:errorcluster)  [unwired: 8 in, 1 out]
      }
    }
    frame Error {
      n190 = call "Synchronize Caller Events.vi"("Module Admin"=w496) -> ("Module Admin out"=w495:refnum<class "Delacor_lib_QMH_Cloneable Module Admin.lvclass">)  [unwired: 9 in, 1 out]
      n191 = property class="Mod Admin"(reference=w495) -> ("Accessors:Module ID"=w494:i32)  [unwired: 1 in, 2 out]
      n192 = call-dynamic "Delacor_lib_QMH_Release Message Queue.vi"("Message Queue"=w492) -> ()  [unwired: 10 in, 1 out]
      n193 = call-dynamic "Delacor_lib_QMH_Release Message Queue.vi"("Message Queue"=w491) -> ()  [unwired: 10 in, 1 out]
      n194 = call "Module Name--constant.vi"("Module ID"=w494) -> ("Module Name"=w499:string)  [unwired: 10 in]
      n195 = Format Into String(format string="An error occurred during initialization. %s is no longer running.", w499) -> (resulting string=w497:string)  [unwired: 2 in, 1 out]
      n196 = call "Error Reported.vi"("Additional Information"=w497, "Error"=w500, "Module ID"=w494) -> ()  [unwired: 8 in, 1 out]
    }
  }
  n197 = Merge Errors(w24, w23) -> (w25:errorcluster)
  n198 = call "Close Module.vi"("error in (no error)"=w25, "Wait for stop?"=w15, "Module Admin in"=w17) -> ("error out"=w9:errorcluster, "External Launch"=w13:bool, "Module Admin out"=w16:refnum<class "Delacor_lib_QMH_Cloneable Module Admin.lvclass">)  [unwired: 6 in]
  n199 = Unregister For Events(event registration refnum=w7, error in=w9) -> (error out=w8:errorcluster)
  n200 = Unregister For Events(event registration refnum=w21, error in=w8) -> (error out=w14:errorcluster)
  "error out" <- w14
  n201 = local write "Module Admin"(w16) -> ()
  n202 = case "External Launch?" shown="True" w13 {
    tunnel: w14 -> [_ w502]
    frame False {
    }
    frame True {
      n203 = case shown="No Error" w502 {
        frame No Error {
          n204 = invoke class="VI" method="FP.Close"() -> ()  [unwired: 3 in, 3 out]
        }
        frame Error {
          n205 = invoke class="VI" method="FP.Open"("Activate"=TRUE ("Activate?")) -> ()  [unwired: 4 in, 5 out]
        }
      }
    }
  }
